vi "Main.vi"() -> ()   [LabVIEW 2015]
uses:
  <vilib>/Instr/_visa.llb/VISA Open Access Mode.ctl
  <vilib>/Instr/_visa.llb/VISA Configure Serial Port (Instr).vi
panel:
  in  "Tab Control":enum32{"Main Program", "Calibration"}(tab)
  out "Voltage8":dbl
  out "Voltage7":dbl
  out "Voltage6":dbl
  out "Voltage5":dbl
  out "Voltage4":dbl
  out "Voltage3":dbl
  out "Voltage2":dbl
  in  "Sampling rate (sample/s)":dbl=10.0
  out "Waveform Chart":T1(graph)
  in  "Current set (mA)":u16[](array[numeric])=[0, 0, 0, 0, 0, 0, 0, 0]
  in  "update curr":bool
  out "Thermometer":i8(slide) scale=10.0..130.0
  out "Temp °C":i8
  in  "VISA resource name":refnum<visa-resource-name>
  in  "relay_1":bool
  in  "relay_2":bool
  in  "relay_3":bool
  in  "relay_4":bool
  in  "relay_5":bool
  in  "relay_6":bool
  in  "relay_7":bool
  out "connected?":bool
  in  "Ch1":bool
  in  "Ch2":bool
  in  "Ch3":bool
  in  "Ch4":bool
  in  "Ch5":bool
  in  "Ch6":bool
  in  "Ch7":bool
  in  "Ch8":bool
  in  "active_ch 1":bool
  in  "active_ch 2":bool
  in  "active_ch 3":bool
  in  "active_ch 4":bool
  in  "active_ch 5":bool
  in  "active_ch 6":bool
  in  "active_ch 7":bool
  in  "active_ch 8":bool
  in  "START":bool
  in  "stop 2":bool
  in  "stop":bool
  out "Voltage1":dbl
  out "sent current code":u16[](array[numeric])
  out "received voltage code":u16[](array[numeric])
  in  "calib_low":u16[](array[numeric]) max=4095 step=1 format="%03x"
  in  "calib_high":u16[](array[numeric]) max=4095 step=1 format="%03x"
  in  "update_eeprom":bool
  out "eeprom_calib_data":u8[](array[numeric]) format="%02x"
  in  "read_calib":bool
  # "Active \nchannels"
  # "6V max"
  # "16V max"
  # "Relays"
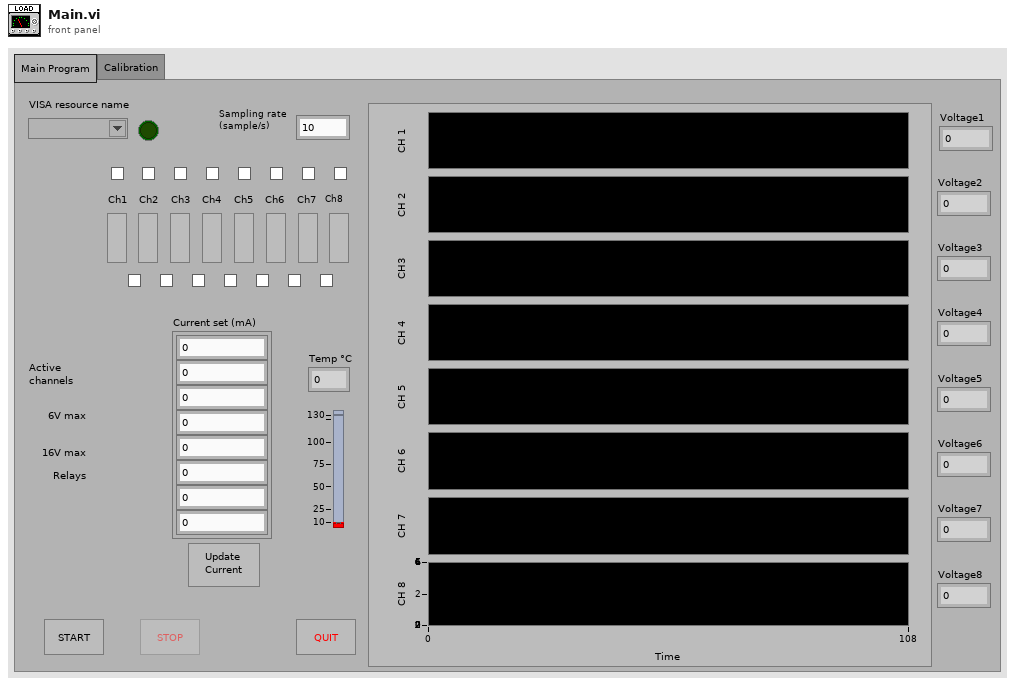
[diagram p1: front panel]
types:
  T1 = cluster{"Command":u16, "Command":u16, "Command":u16, "Command":u16, "Command":u16, "Command":u16, "Command":u16, "Command":u16}
  T2 = enum8{"Enabled", "Disabled", "Disabled and Grayed Out"}
  T3 = typedef "VISA Open Access Mode.ctl" = u32
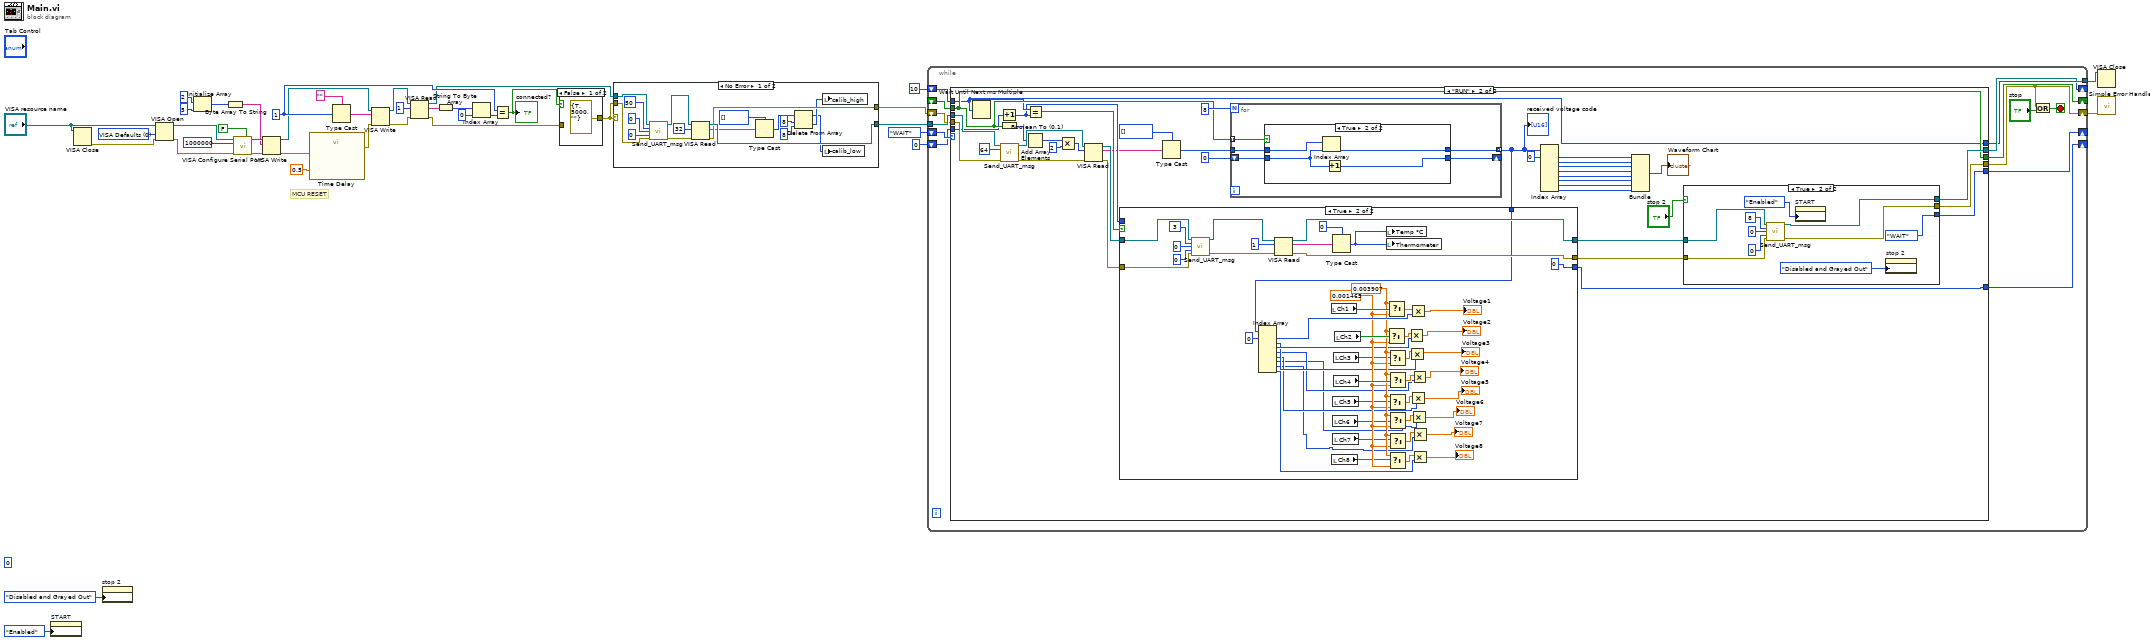
[diagram p0: block diagram]
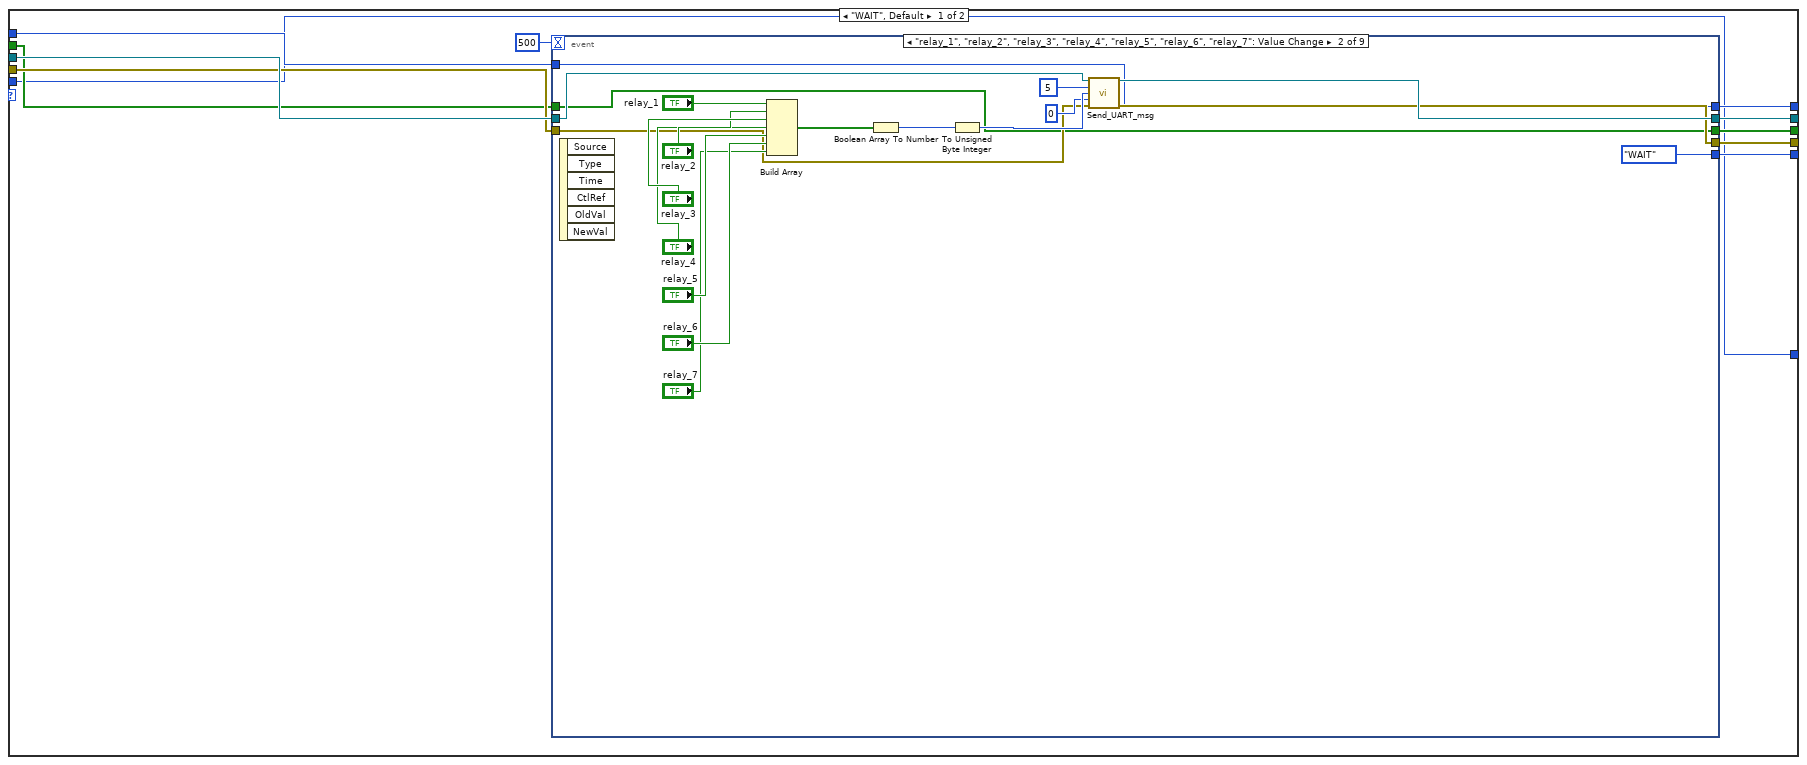
[diagram p3: hidden frame]
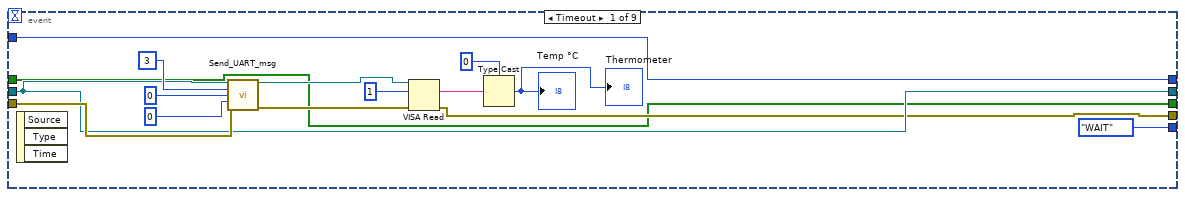
[diagram p4: hidden frame]
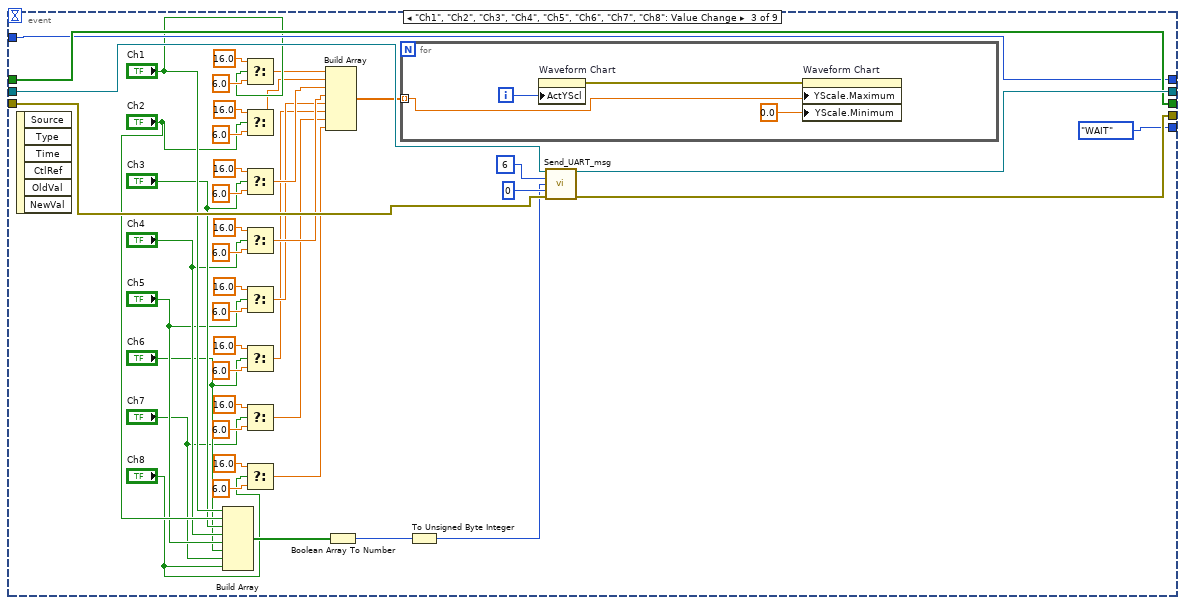
[diagram p5: hidden frame]
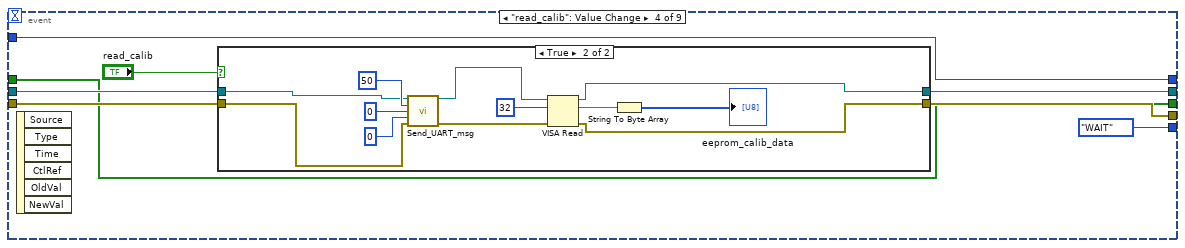
[diagram p6: hidden frame]
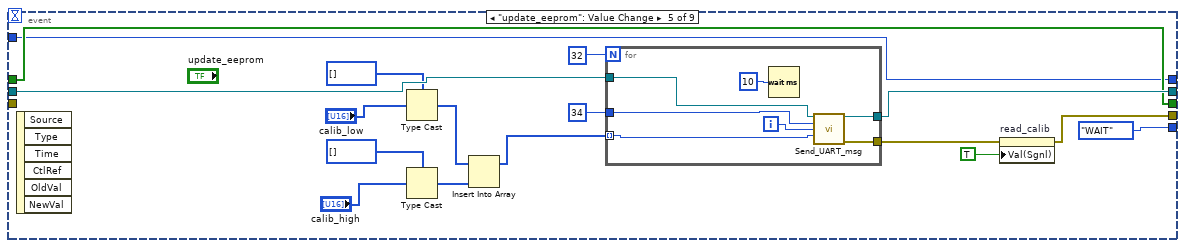
[diagram p8: hidden frame]
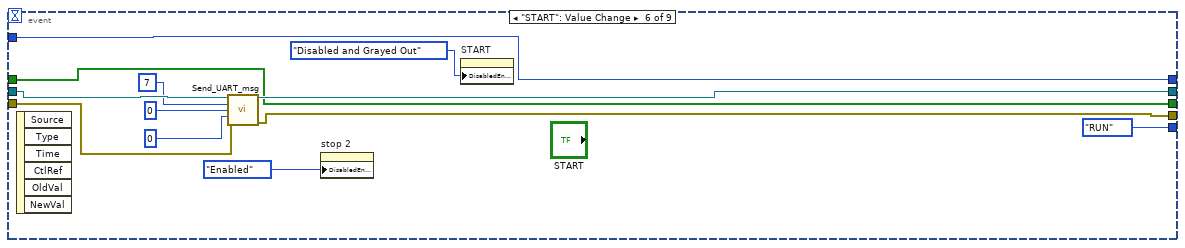
[diagram p9: hidden frame]
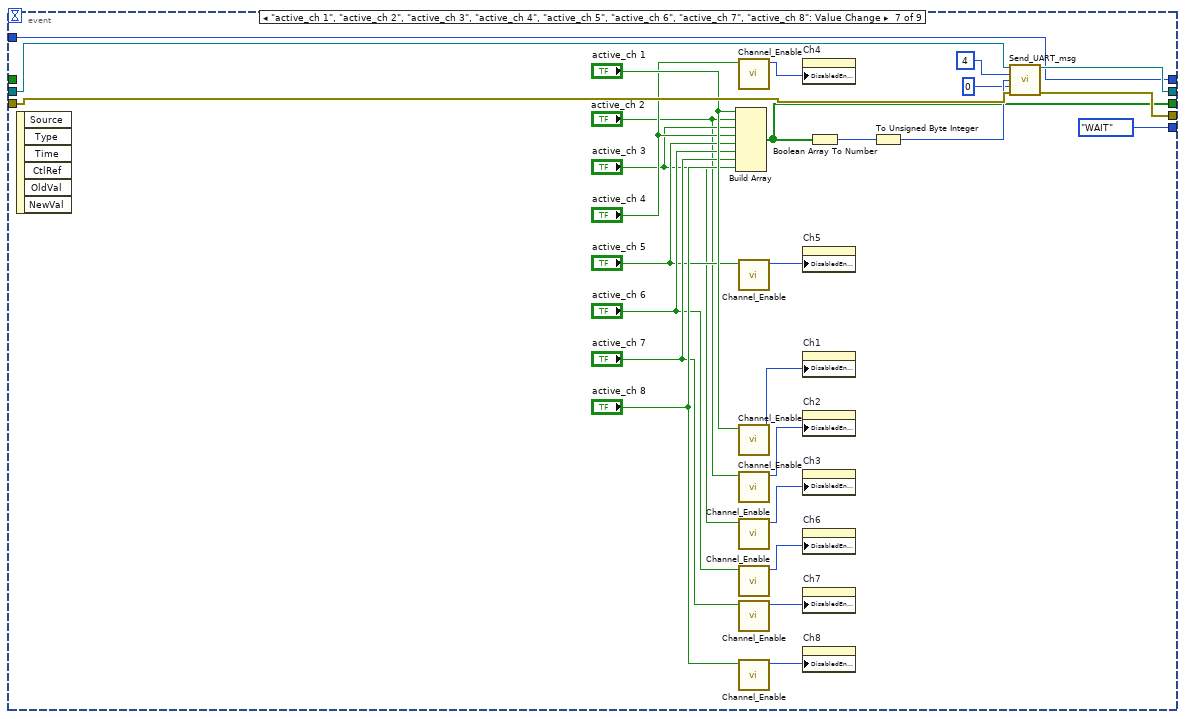
[diagram p10: hidden frame]
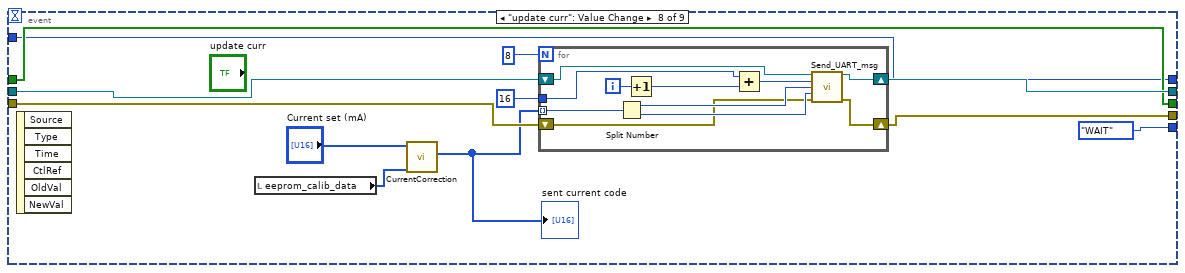
[diagram p11: hidden frame]
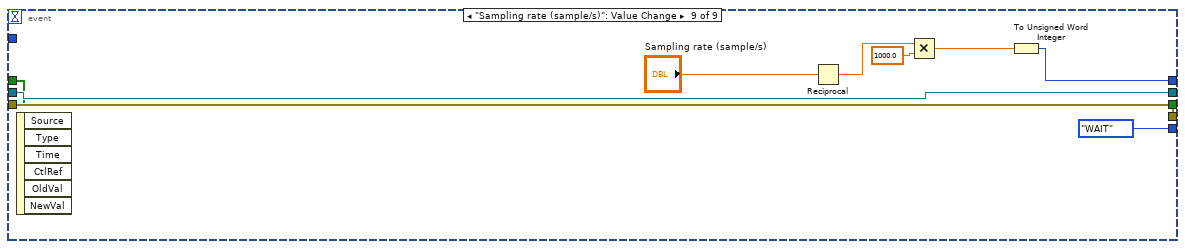
[diagram p12: hidden frame]
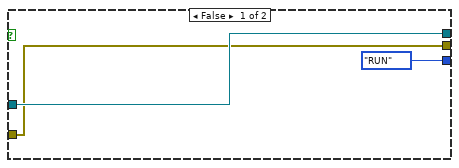
[diagram p14: hidden frame]
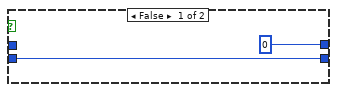
[diagram p15: hidden frame]
diagram:
  (unwired) u8 0
  w23 = T3 0 items=["VISA Defaults"=0, "Exclusive Lock"=1, "Load Configured Settings"=4] ("Access Mode")
  w35 = 1
  # "MCU RESET"
  n1 = property on="START" class="Bool"("DisabledEnum"=T2."Enabled" ("Disabled")) -> ()  [unwired: 2 in, 2 out]
  n2 = VISA Close(VISA resource name="VISA resource name") -> (error out=w20:errorcluster)  [unwired: 1 in]
  n3 = property on="stop 2" class="Bool"("DisabledEnum"=T2."Disabled and Grayed Out" ("Disabled")) -> ()  [unwired: 2 in, 2 out]
  n4 = VISA Open(access mode=w23, error in (no error)=w20, VISA resource name="VISA resource name") -> (VISA resource name=w25:refnum<visa-resource-name>, error out=w24:errorcluster)  [unwired: 2 in]
  n5 = Initialize Array(u8 2 ("element"), 5 ("dimension size")) -> (w17:u8[])
  n6 = Byte Array To String(unsigned byte array=w17) -> (string=w14:string)
  n7 = call-poly "VISA Configure Serial Port"("VISA resource name"=w25, "Enable Termination\nChar (T)"=FALSE ("Enable Termination\nChar (T)"), "baud rate (9600)"=u32 1000000, "error in (no error)"=w24) -> ("VISA resource name out"=w15:refnum<visa-resource-name>, "error out"=w16:errorcluster)  [unwired: 10 in]
  n8 = VISA Write(VISA resource name=w15, write buffer=w14, error in (no error)=w16) -> (VISA resource name out=w10:refnum<visa-resource-name>, error out=w12:errorcluster)  [unwired: 1 out]
  n9 = call "Time Delay"("error in (no error)"=w12, "Delay Time (s)"=0.5) -> ("error out"=w11:errorcluster)  [unwired: 9 in]
  n10 = Type Cast(type="", x=w35) -> (*(type *) &x=w40:string)
  n11 = VISA Write(VISA resource name=w10, write buffer=w40, error in (no error)=w11) -> (VISA resource name out=w37:refnum<visa-resource-name>, error out=w36:errorcluster)  [unwired: 1 out]
  n12 = VISA Read(VISA resource name=w37, byte count=u32 1, error in (no error)=w36) -> (VISA resource name out=w5:refnum<visa-resource-name>, read buffer=w30:string, error out=w34:errorcluster)  [unwired: 1 out]
  n13 = String To Byte Array(string=w30) -> (unsigned byte array=w28:u8[])
  n14 = Index Array(array=w28, index=0) -> (element=w26:u8)
  n15 = Equal?(x=w35, y=w26) -> (x = y?=w29:bool)
  "connected?" <- w29
  n16 = case shown="False" w29 {
    tunnel: [errorcluster {"status"=TRUE, "code"=5000, "source"=""} ("error constant") w42] -> w3
    tunnel: w34 -> [_ w42]
    frame False {
    }
    frame True {
    }
  }
  n17 = case shown="No Error" w3 {
    tunnel: w3 -> [w56 w60]
    tunnel: w5 -> [w55 w61]
    tunnel: [w51 w61] -> w4
    tunnel: [w50 w60] -> w6
    frame No Error {
      n18 = call "Send_UART_msg.vi"("VISA Refnum in"=w55, "Command"=u8 50, "Data 1"=u8 0, "Data 2"=u8 0, "error in (no error)"=w56) -> ("VISA Refnum out"=w53:refnum<visa-resource-name>, "error out"=w54:errorcluster)  [unwired: 8 in, 1 out]
      n19 = VISA Read(VISA resource name=w53, byte count=u32 32, error in (no error)=w54) -> (VISA resource name out=w51:refnum<visa-resource-name>, read buffer=w45:string, error out=w50:errorcluster)  [unwired: 1 out]
      n20 = Type Cast(type=u16[] [], x=w45) -> (*(type *) &x=w44:u16[])
      n21 = Delete From Array(array=w44, length=8, index=8) -> (deleted portion=w47:u16[], array with subset deleted=w46:u16[])
      n22 = local write "calib_high"(w47) -> ()
      n23 = local write "calib_low"(w46) -> ()
    }
    frame Error {
    }
  }
  n24 = while {
    shift-right: [w71] -> w9
    shift-left: w6 -> [w74]
    tunnel: w4 -> [w75]
    shift-right: [w68] -> _
    shift-left: enum16{"WAIT", "RUN", "LOST"}."WAIT" -> [w69]
    tunnel: [w73] -> w22
    shift-right: [w66] -> _
    shift-left: _ -> [w67]
    shift-right: [w65] -> _
    shift-left: u16 10 -> [w64]
    shift-right: [w62] -> _
    shift-left: 0 -> [w63]
    stop <- w70 stop-if-true
    n25 = case shown="\"RUN\"" w69 {
      tunnel: w75 -> [w86 w321]
      tunnel: w74 -> [w85 w320]
      tunnel: [w84 w324] -> w73
      tunnel: [w83 w323] -> w71
      tunnel: [w81 w325] -> w68
      tunnel: w67 -> [w80 w306]
      tunnel: [w79 w306] -> w66
      tunnel: [w78 w301] -> w65
      tunnel: w64 -> [w77 w301]
      tunnel: w63 -> [w76 w302]
      tunnel: [w76 w294] -> w62
      frame "WAIT", Default {
        n26 = event shown="[1] \"relay_1\", \"relay_2\", \"relay_3\", \"relay_4\", \"relay_5\", \"relay_6\", \"relay_7\": Value Change" {
          selector: _ -> [_ _ _ _ _ _ _ _ _]
          dyn-events: _ -> [_ _ _ _ _ _ _ _ _]
          timeout: 500 -> [_ _ _ _ _ _ _ _ _]
          tunnel: w86 -> [w94 w108 w159 w176 w208 w227 w253 w260 w281]
          tunnel: w85 -> [w101 w106 w162 w177 _ w226 w252 w264 w280]
          tunnel: [w93 w105 w161 w174 w203 w222 w247 w263 w280] -> w83
          tunnel: [w94 w107 w160 w175 w205 w220 w248 w261 w281] -> w84
          tunnel: [enum16{"WAIT", "RUN", "LOST"}."WAIT" enum16{"WAIT", "RUN", "LOST"}."WAIT" enum16{"WAIT", "RUN", "LOST"}."WAIT" enum16{"WAIT", "RUN", "LOST"}."WAIT" enum16{"WAIT", "RUN", "LOST"}."WAIT" enum16{"WAIT", "RUN", "LOST"}."RUN" enum16{"WAIT", "RUN", "LOST"}."WAIT" enum16{"WAIT", "RUN", "LOST"}."WAIT" enum16{"WAIT", "RUN", "LOST"}."WAIT"] -> w81
          tunnel: w80 -> [w91 w103 w155 w171 w193 w217 _ w259 w278]
          tunnel: [w91 w103 w155 w171 w193 w217 w245 w259 w278] -> w79
          tunnel: [w90 w102 w154 w170 w192 w216 w228 w258 w283] -> w78
          tunnel: w77 -> [w90 w102 w154 w170 w192 w216 w228 w258 _]
          event Timeout {
            n27 = event-data() -> ()  [unwired: 1 in, 3 out]
            n28 = call "Send_UART_msg.vi"("VISA Refnum in"=w94, "Command"=u8 3, "Data 1"=u8 0, "Data 2"=u8 0, "error in (no error)"=w101) -> ("VISA Refnum out"=w97:refnum<visa-resource-name>, "error out"=w95:errorcluster)  [unwired: 8 in, 1 out]
            n29 = VISA Read(VISA resource name=w97, byte count=u32 1, error in (no error)=w95) -> (read buffer=w89:string, error out=w93:errorcluster)  [unwired: 2 out]
            n30 = Type Cast(type=i8 0, x=w89) -> (*(type *) &x=→"Thermometer" →"Temp °C":i8)
          }
          event "relay_1", "relay_2", "relay_3", "relay_4", "relay_5", "relay_6", "relay_7": Value Change {
            n31 = event-data() -> ()  [unwired: 1 in, 6 out]
            n32 = Build Array("relay_1", "relay_2", "relay_3", "relay_4", "relay_5", "relay_6", "relay_7") -> (w113:bool[])
            n33 = Boolean Array To Number(Boolean array=w113) -> (number=w112:u32)
            n34 = To Unsigned Byte Integer(number=w112) -> (unsigned 8bit integer=w111:u8)
            n35 = call "Send_UART_msg.vi"("VISA Refnum in"=w108, "Command"=u8 5, "Data 1"=w111, "Data 2"=u8 0, "error in (no error)"=w106) -> ("VISA Refnum out"=w107:refnum<visa-resource-name>, "error out"=w105:errorcluster)  [unwired: 8 in, 1 out]
          }
          event "Ch1", "Ch2", "Ch3", "Ch4", "Ch5", "Ch6", "Ch7", "Ch8": Value Change {
            n36 = event-data() -> ()  [unwired: 1 in, 6 out]
            n37 = Build Array("Ch1", "Ch2", "Ch3", "Ch4", "Ch5", "Ch6", "Ch7", "Ch8") -> (w156:bool[])
            n38 = Select(t=16.0, s="Ch1", f=6.0) -> (s? t:f=w129:dbl)
            n39 = Select(t=16.0, s="Ch2", f=6.0) -> (s? t:f=w128:dbl)
            n40 = Select(t=16.0, s="Ch3", f=6.0) -> (s? t:f=w127:dbl)
            n41 = Select(t=16.0, s="Ch4", f=6.0) -> (s? t:f=w126:dbl)
            n42 = Select(t=16.0, s="Ch5", f=6.0) -> (s? t:f=w125:dbl)
            n43 = Select(t=16.0, s="Ch6", f=6.0) -> (s? t:f=w124:dbl)
            n44 = Select(t=16.0, s="Ch7", f=6.0) -> (s? t:f=w123:dbl)
            n45 = Select(t=16.0, s="Ch8", f=6.0) -> (s? t:f=w122:dbl)
            n46 = Build Array(w129, w128, w127, w126, w125, w124, w123, w122) -> (w121:dbl[])
            n47 = Boolean Array To Number(Boolean array=w156) -> (number=w165:u32)
            n48 = for {
              tunnel: w121 -> [w166] mode=indexing
              i -> [w168]
              n49 = property on="Waveform Chart" class="WFChart (strict)"("ActYScl"=w168) -> (error out=w167:errorcluster)  [unwired: 2 in, 1 out]
              n50 = property on="Waveform Chart" class="WFChart (strict)"(error in=w167, "YScale.Maximum"=w166, "YScale.Minimum"=0.0 ("Y Scale.Range:Minimum")) -> ()  [unwired: 1 in, 2 out]
            }
            n51 = To Unsigned Byte Integer(number=w165) -> (unsigned 8bit integer=w157:u8)
            n52 = call "Send_UART_msg.vi"("VISA Refnum in"=w159, "Command"=u8 6, "Data 1"=w157, "Data 2"=u8 0, "error in (no error)"=w162) -> ("VISA Refnum out"=w160:refnum<visa-resource-name>, "error out"=w161:errorcluster)  [unwired: 8 in, 1 out]
          }
          event "read_calib": Value Change {
            n53 = event-data() -> ()  [unwired: 1 in, 6 out]
            n54 = case shown="True" "read_calib" {
              tunnel: w177 -> [w178 w188]
              tunnel: w176 -> [w179 w187]
              tunnel: [w179 w183] -> w175
              tunnel: [w178 w182] -> w174
              frame False {
              }
              frame True {
                n55 = call "Send_UART_msg.vi"("VISA Refnum in"=w187, "Command"=u8 50, "Data 1"=u8 0, "Data 2"=u8 0, "error in (no error)"=w188) -> ("VISA Refnum out"=w185:refnum<visa-resource-name>, "error out"=w186:errorcluster)  [unwired: 8 in, 1 out]
                n56 = VISA Read(VISA resource name=w185, byte count=u32 32, error in (no error)=w186) -> (VISA resource name out=w183:refnum<visa-resource-name>, read buffer=w181:string, error out=w182:errorcluster)  [unwired: 1 out]
                n57 = String To Byte Array(string=w181) -> (unsigned byte array=→"eeprom_calib_data":u8[])
              }
            }
          }
          event "update_eeprom": Value Change {
            n58 = event-data() -> ()  [unwired: 1 in, 6 out]
            n59 = Type Cast(type=u8[] [], x="calib_low") -> (*(type *) &x=w197:u8[])
            n60 = Type Cast(type=u8[] [], x="calib_high") -> (*(type *) &x=w196:u8[])
            n61 = Insert Into Array(array=w197, new element=w196) -> (w198:u8[])  [unwired: 1 in]
            n62 = for {
              N: 32 -> [_]
              tunnel: w208 -> [w215]
              tunnel: u8 34 -> [w214]
              tunnel: w198 -> [w212] mode=indexing
              tunnel: [w211] -> w205
              tunnel: [w210] -> w204
              i -> [w213]
              n63 = Wait (ms)(milliseconds to wait=u32 10 ("millisecond multiple")) -> ()  [unwired: 1 out]
              n64 = call "Send_UART_msg.vi"("VISA Refnum in"=w215, "Command"=w214, "Data 1"=w213, "Data 2"=w212) -> ("VISA Refnum out"=w211:refnum<visa-resource-name>, "error out"=w210:errorcluster)  [unwired: 9 in, 1 out]
            }
            n65 = property on="read_calib" class="Bool (strict)"(error in=w204, "Val(Sgnl)"=TRUE ("Value (Signaling)")) -> (error out=w203:errorcluster)  [unwired: 1 in, 1 out]
          }
          event "START": Value Change {
            n66 = event-data() -> ()  [unwired: 1 in, 6 out]
            n67 = call "Send_UART_msg.vi"("VISA Refnum in"=w227, "Command"=u8 7, "Data 1"=u8 0, "Data 2"=u8 0, "error in (no error)"=w226) -> ("VISA Refnum out"=w220:refnum<visa-resource-name>, "error out"=w222:errorcluster)  [unwired: 8 in, 1 out]
            n68 = property on="stop 2" class="Bool"("DisabledEnum"=T2."Enabled" ("Disabled")) -> ()  [unwired: 2 in, 2 out]
            n69 = property on="START" class="Bool"("DisabledEnum"=T2."Disabled and Grayed Out" ("Disabled")) -> ()  [unwired: 2 in, 2 out]
          }
          event "active_ch 1", "active_ch 2", "active_ch 3", "active_ch 4", "active_ch 5", "active_ch 6", "active_ch 7", "active_ch 8": Value Change {
            n70 = event-data() -> ()  [unwired: 1 in, 6 out]
            n71 = Build Array("active_ch 1", "active_ch 2", "active_ch 3", "active_ch 4", "active_ch 5", "active_ch 6", "active_ch 7", "active_ch 8") -> (w245:bool[])
            n72 = call "Channel_Enable.vi"("active_ch 1"="active_ch 4") -> ("Disabled"=w240:T2)  [unwired: 10 in]
            n73 = call "Channel_Enable.vi"("active_ch 1"="active_ch 5") -> ("Disabled"=w239:T2)  [unwired: 10 in]
            n74 = call "Channel_Enable.vi"("active_ch 1"="active_ch 1") -> ("Disabled"=w244:T2)  [unwired: 10 in]
            n75 = call "Channel_Enable.vi"("active_ch 1"="active_ch 2") -> ("Disabled"=w242:T2)  [unwired: 10 in]
            n76 = call "Channel_Enable.vi"("active_ch 1"="active_ch 3") -> ("Disabled"=w241:T2)  [unwired: 10 in]
            n77 = call "Channel_Enable.vi"("active_ch 1"="active_ch 6") -> ("Disabled"=w238:T2)  [unwired: 10 in]
            n78 = call "Channel_Enable.vi"("active_ch 1"="active_ch 7") -> ("Disabled"=w237:T2)  [unwired: 10 in]
            n79 = call "Channel_Enable.vi"("active_ch 1"="active_ch 8") -> ("Disabled"=w236:T2)  [unwired: 10 in]
            n80 = property on="Ch4" class="Bool (strict)"("DisabledEnum"=w240) -> ()  [unwired: 2 in, 2 out]
            n81 = property on="Ch5" class="Bool (strict)"("DisabledEnum"=w239) -> ()  [unwired: 2 in, 2 out]
            n82 = property on="Ch1" class="Bool (strict)"("DisabledEnum"=w244) -> ()  [unwired: 2 in, 2 out]
            n83 = property on="Ch2" class="Bool (strict)"("DisabledEnum"=w242) -> ()  [unwired: 2 in, 2 out]
            n84 = property on="Ch3" class="Bool (strict)"("DisabledEnum"=w241) -> ()  [unwired: 2 in, 2 out]
            n85 = property on="Ch6" class="Bool (strict)"("DisabledEnum"=w238) -> ()  [unwired: 2 in, 2 out]
            n86 = property on="Ch7" class="Bool (strict)"("DisabledEnum"=w237) -> ()  [unwired: 2 in, 2 out]
            n87 = property on="Ch8" class="Bool (strict)"("DisabledEnum"=w236) -> ()  [unwired: 2 in, 2 out]
            n88 = Boolean Array To Number(Boolean array=w245) -> (number=w254:u32)
            n89 = To Unsigned Byte Integer(number=w254) -> (unsigned 8bit integer=w251:u8)
            n90 = call "Send_UART_msg.vi"("VISA Refnum in"=w253, "Command"=u8 4, "Data 1"=w251, "Data 2"=u8 0, "error in (no error)"=w252) -> ("VISA Refnum out"=w248:refnum<visa-resource-name>, "error out"=w247:errorcluster)  [unwired: 8 in, 1 out]
          }
          event "update curr": Value Change {
            n91 = event-data() -> ()  [unwired: 1 in, 6 out]
            n92 = local read "eeprom_calib_data"() -> (w256:u8[])
            n93 = call "CurrentCorrection.vi"("Calib_data"=w256, "Current_in_mA"="Current set (mA)") -> ("Correct_Code"=w255:u16[])  [unwired: 9 in]
            "sent current code" <- w255
            n94 = for {
              N: 8 -> [_]
              tunnel: w255 -> [w277] mode=indexing
              tunnel: u8 16 ("Command") -> [w272]
              shift-right: [w270] -> w263
              shift-left: w264 -> [w269]
              shift-right: [w268] -> w261
              shift-left: w260 -> [w267]
              i -> [w274]
              n95 = Split Number(x=w277) -> (hi(x)=w276:u8, lo(x)=w275:u8)
              n96 = Increment(x=w274) -> (x+1=w273:i32)
              n97 = Add(x=w272, y=w273) -> (x+y=w271:i32)
              n98 = call "Send_UART_msg.vi"("VISA Refnum in"=w267, "Command"=w271, "Data 1"=w276, "Data 2"=w275, "error in (no error)"=w269) -> ("VISA Refnum out"=w268:refnum<visa-resource-name>, "error out"=w270:errorcluster)  [unwired: 8 in, 1 out]
            }
          }
          event "Sampling rate (sample/s)": Value Change {
            n99 = event-data() -> ()  [unwired: 1 in, 6 out]
            n100 = Reciprocal(x="Sampling rate (sample/s)") -> (1/x=w282:dbl)
            n101 = Multiply(x=w282, y=1000.0) -> (x*y=w284:dbl)
            n102 = To Unsigned Word Integer(number=w284) -> (unsigned 16bit integer=w283:u16)
          }
        }
      }
      frame "RUN" {
        n103 = Wait Until Next ms Multiple(millisecond multiple=w301) -> ()  [unwired: 1 out]
        n104 = Boolean To (0,1)(Boolean=w306) -> (0, 1=w317:i16[])
        n105 = Increment(x=w302) -> (x+1=w295:i32)
        n106 = call "Send_UART_msg.vi"("VISA Refnum in"=w321, "Command"=u8 64, "error in (no error)"=w320) -> ("VISA Refnum out"=w319:refnum<visa-resource-name>, "error out"=w318:errorcluster)  [unwired: 10 in, 1 out]
        n107 = Equal?(x=w301, y=w295) -> (x = y?=w299:bool)
        n108 = Add Array Elements(numeric array=w317) -> (sum=w293:i16)
        n109 = Multiply(x=w293, y=i16 2) -> (x*y=w291:i16)
        n110 = VISA Read(VISA resource name=w319, byte count=w291, error in (no error)=w318) -> (VISA resource name out=w298:refnum<visa-resource-name>, read buffer=w290:string, error out=w300:errorcluster)  [unwired: 1 out]
        n111 = Type Cast(type=u16[] [], x=w290) -> (*(type *) &x=w288:u16[])
        n112 = for {
          N: 8 -> [_]
          tunnel: w306 -> [w396] mode=indexing
          tunnel: w288 -> [w393]
          tunnel: [w395] -> w287 mode=indexing
          shift-right: [w392] -> _
          shift-left: 0 -> [w394]
          n113 = case shown="True" w396 {
            tunnel: [u16 0 w401] -> w395
            tunnel: w394 -> [w397 w399]
            tunnel: w393 -> [_ w402]
            tunnel: [w397 w400] -> w392
            frame False {
            }
            frame True {
              n114 = Index Array(array=w402, index=w399) -> (element=w401:u16)
              n115 = Increment(x=w399) -> (x+1=w400:i32)
            }
          }
        }
        "received voltage code" <- w287
        n116 = case shown="True" w299 {
          tunnel: w300 -> [w327 w371]
          tunnel: w298 -> [w328 w370]
          tunnel: [w328 w369] -> w297
          tunnel: [w327 w366] -> w296
          tunnel: w295 -> [w326 _]
          tunnel: [w326 0] -> w294
          tunnel: w287 -> [_ w362]
          frame False {
          }
          frame True {
            w354 = 0.001465 ("x")
            w355 = 0.003907 ("x")
            n117 = call "Send_UART_msg.vi"("VISA Refnum in"=w370, "Command"=u8 3, "Data 1"=u8 0, "Data 2"=u8 0, "error in (no error)"=w371) -> ("VISA Refnum out"=w375:refnum<visa-resource-name>, "error out"=w373:errorcluster)  [unwired: 8 in, 1 out]
            n118 = Index Array(array=w362, index #1=0 ("index")) -> (element #1=w357:u16, element #2=w342:u16, element #3=w341:u16, element #4=w340:u16, element #5=w339:u16, element #6=w338:u16, element #7=w337:u16, element #8=w336:u16)  [unwired: 7 in]
            n119 = VISA Read(VISA resource name=w375, byte count=u32 1, error in (no error)=w373) -> (VISA resource name out=w369:refnum<visa-resource-name>, read buffer=w372:string, error out=w366:errorcluster)  [unwired: 1 out]
            n120 = local read "Ch1"() -> (w359:bool)
            n121 = local read "Ch8"() -> (w349:bool)
            n122 = local read "Ch6"() -> (w351:bool)
            n123 = Type Cast(type=u8 0, x=w372) -> (*(type *) &x=w367:u8)
            n124 = local read "Ch5"() -> (w352:bool)
            n125 = local read "Ch7"() -> (w350:bool)
            n126 = local read "Ch3"() -> (w353:bool)
            n127 = local read "Ch4"() -> (w363:bool)
            n128 = local read "Ch2"() -> (w364:bool)
            n129 = local write "Temp °C"(w367) -> ()
            n130 = local write "Thermometer"(w367) -> ()
            n131 = Select(t=w355, s=w364, f=w354) -> (s? t:f=w356:dbl)
            n132 = Select(t=w355, s=w359, f=w354) -> (s? t:f=w360:dbl)
            n133 = Select(t=w355, s=w353, f=w354) -> (s? t:f=w343:dbl)
            n134 = Select(t=w355, s=w352, f=w354) -> (s? t:f=w345:dbl)
            n135 = Select(t=w355, s=w349, f=w354) -> (s? t:f=w348:dbl)
            n136 = Select(t=w355, s=w363, f=w354) -> (s? t:f=w344:dbl)
            n137 = Select(t=w355, s=w351, f=w354) -> (s? t:f=w346:dbl)
            n138 = Select(t=w355, s=w350, f=w354) -> (s? t:f=w347:dbl)
            n139 = Multiply(x=w356, y=w342) -> (x*y=→"Voltage2":dbl)
            n140 = Multiply(x=w343, y=w341) -> (x*y=→"Voltage3":dbl)
            n141 = Multiply(x=w360, y=w357) -> (x*y=→"Voltage1":dbl)
            n142 = Multiply(x=w345, y=w339) -> (x*y=→"Voltage5":dbl)
            n143 = Multiply(x=w346, y=w338) -> (x*y=→"Voltage6":dbl)
            n144 = Multiply(x=w344, y=w340) -> (x*y=→"Voltage4":dbl)
            n145 = Multiply(x=w347, y=w337) -> (x*y=→"Voltage7":dbl)
            n146 = Multiply(x=w348, y=w336) -> (x*y=→"Voltage8":dbl)
          }
        }
        n147 = Index Array(array=w287, index #1=0 ("index")) -> (element #1=w308:u16, element #2=w309:u16, element #3=w310:u16, element #4=w311:u16, element #5=w312:u16, element #6=w313:u16, element #7=w314:u16, element #8=w315:u16)  [unwired: 7 in]
        n148 = Bundle("Command"=w308, "Command"=w309, "Command"=w310, "Command"=w311, "Command"=w312, "Command"=w313, "Command"=w314, "Command"=w315) -> (→"Waveform Chart":T1)  [unwired: 1 in]
        n149 = case shown="True" "stop 2" {
          tunnel: [enum16{"WAIT", "RUN", "LOST"}."RUN" enum16{"WAIT", "RUN", "LOST"}."WAIT"] -> w325
          tunnel: [w380 w390] -> w324
          tunnel: [w379 w389] -> w323
          tunnel: w296 -> [w379 w388]
          tunnel: w297 -> [w380 w387]
          frame False {
          }
          frame True {
            n150 = call "Send_UART_msg.vi"("VISA Refnum in"=w387, "Command"=u8 8, "Data 1"=u8 0, "Data 2"=u8 0, "error in (no error)"=w388) -> ("VISA Refnum out"=w390:refnum<visa-resource-name>, "error out"=w389:errorcluster)  [unwired: 8 in, 1 out]
            n151 = property on="START" class="Bool"("DisabledEnum"=T2."Enabled" ("Disabled")) -> ()  [unwired: 2 in, 2 out]
            n152 = property on="stop 2" class="Bool"("DisabledEnum"=T2."Disabled and Grayed Out" ("Disabled")) -> ()  [unwired: 2 in, 2 out]
          }
        }
      }
    }
    n153 = Or(x=w71, y="stop") -> (x .or. y?=w70:bool)
  }
  n154 = VISA Close(VISA resource name=w22) -> ()  [unwired: 1 in, 1 out]
  n155 = call <vilib>:"Simple Error Handler.vi"("error in (no error)"=w9) -> ()  [unwired: 4 in, 5 out]
